vi "Esercitazione 4 - Esercizio per casa, numero primo.vi"() -> ()   [LabVIEW 2018]
panel:
  out "Primo":bool
  in  "Numeric":i32
  # "Dato un numero in INPUT, verificare che sia un numero primo"
  # "meglio usare un while esterno comunque"
  # "divisibile per \nse stesso e 1"
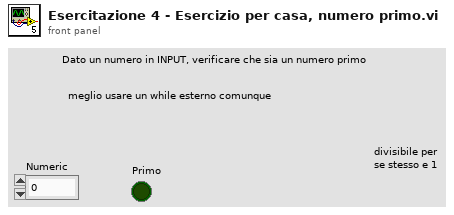
[diagram p1: front panel]
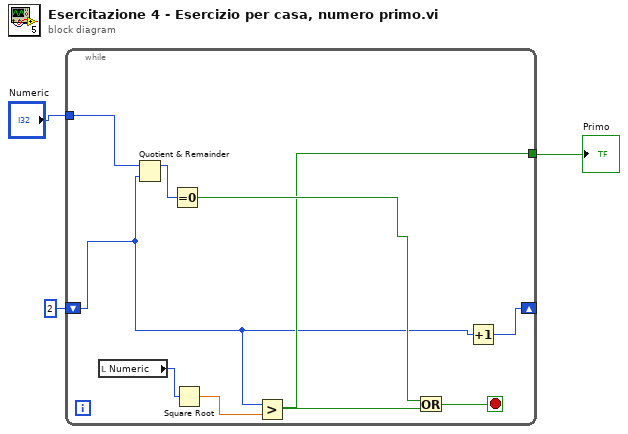
[diagram p0: block diagram]
diagram:
  n1 = while {
    shift-right: [w10] -> _
    shift-left: 2 -> [w6]
    tunnel: [w7] -> w1
    tunnel: "Numeric" -> [w11]
    stop <- w8 stop-if-true
    n2 = local read "Numeric"() -> (w4:i32)
    n3 = Quotient & Remainder(x=w11, y=w6) -> (x-y*floor(x/y)=w12:i32)  [unwired: 1 out]
    n4 = Equal To 0?(x=w12) -> (x = 0?=w9:bool)
    n5 = Square Root(x=w4) -> (sqrt(x)=w5:dbl)
    n6 = Greater?(x=w6, y=w5) -> (0:w7:bool)
    n7 = Or(x=w9, y=w7) -> (x .or. y?=w8:bool)
    n8 = Increment(x=w6) -> (x+1=w10:i32)
  }
  "Primo" <- w1
